vi "stopTask.vi"() -> ()   [LabVIEW 2010, in "pdbm_test_system.lvlib"]
uses:
  pdbm_test_system.lvlib
panel:
  in  "error in (no error)":errorcluster
  in  "ItemName":string
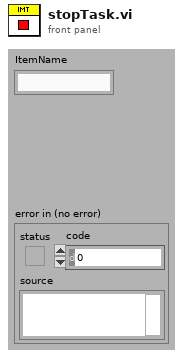
[diagram p1: front panel]
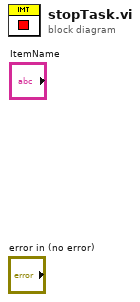
[diagram p0: block diagram]
diagram:
